vi "AIT 664 - Read incoming message data.vi"(0 "Driver Data":T1 {"Num Bits" min=1 max=32}, 5 "Default Msg Data":u8[](array[numeric]), 11 "error in (no error)":errorcluster) -> (4 "Values":dbl[](array[numeric]), 15 "error out":errorcluster)   [LabVIEW 2013, in "AIT 664 Custom Device.lvlib"]
doc: "Given channel definition convert U8 data from AIT 664 card to double array that can then be sent to Veristand"
uses:
  AIT 664 Custom Device.lvlib
  RT Controls/AIT 664 - Driver Data.ctl
  Controls and Global/Start Bit.ctl
  Controls and Global/Number of Bits.ctl
  System Explorer/Controls/664 -Param.ctl
  <vilib>/NI Veristand/Custom Device Tools/Custom Device Utility Library/Custom Device Utility Library.lvlib
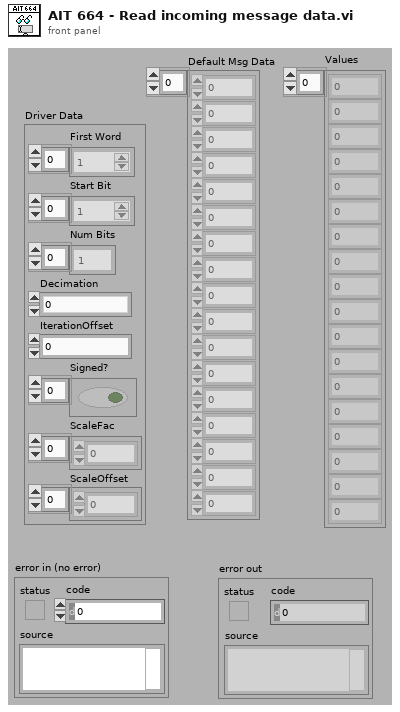
[diagram p1: front panel]
types:
  T1 = typedef "AIT 664 Custom Device.lvlib/AIT 664 - Driver Data.ctl" = cluster{"First Word":T2[], "Start Bit":T2[], "Num Bits":T3[], "Decimation":i32, "IterationOffset":i32, "Signed?":bool[], "ScaleFac":dbl[], "ScaleOffset":dbl[]}
  T2 = typedef "AIT 664 Custom Device.lvlib/Start Bit.ctl" = i32
  T3 = typedef "AIT 664 Custom Device.lvlib/Number of Bits.ctl" = i32
  T4 = typedef "AIT 664 Custom Device.lvlib/664 -Param.ctl" = cluster{"name":string, "firstByte":i32, "startBit":i32, "numberBits":i32, "scaleFactor":dbl, "scaleOffset":dbl, "signed":bool}
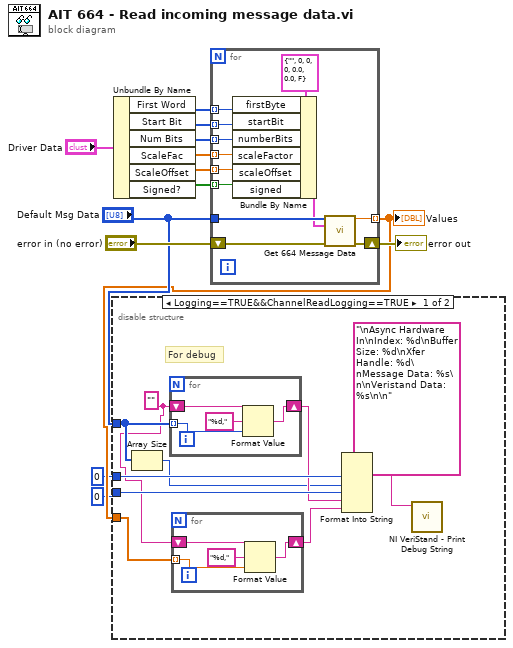
[diagram p0: block diagram]
diagram:
  n1 = Unbundle By Name("Driver Data") -> ("First Word"=w11:T2[], "Start Bit"=w10:T2[], "Num Bits"=w9:T3[], "ScaleFac"=w8:dbl[], "ScaleOffset"=w7:dbl[], "Signed?"=w6:bool[])
  n2 = for {
    tunnel: "Default Msg Data" -> [w25]
    tunnel: w11 -> [w22] mode=indexing
    tunnel: w10 -> [w21] mode=indexing
    tunnel: w9 -> [w20] mode=indexing
    tunnel: w8 -> [w19] mode=indexing
    tunnel: w7 -> [w18] mode=indexing
    tunnel: w6 -> [w17] mode=indexing
    tunnel: [w15] -> w3 mode=indexing
    shift-right: [w14] -> w5
    shift-left: "error in (no error)" -> [w24]
    n3 = Bundle By Name(cluster=T4 {"name"="", "firstByte"=0, "startBit"=0, "numberBits"=0, "scaleFactor"=0.0, "scaleOffset"=0.0, "signed"=FALSE} ("1553 Parameter"), "firstByte"=w22, "startBit"=w21, "numberBits"=w20, "scaleFactor"=w19, "scaleOffset"=w18, "signed"=w17) -> (w16:T4)
    n4 = call "Get 664 Message Data.vi"("MSG DATA"=w25, "664 Parameter"=w16, "error in (no error)"=w24) -> ("Value"=w15:dbl, "error out"=w14:errorcluster)  [unwired: 11 in]
  }
  "error out" <- w5
  "Values" <- w3
  n5 = disable-structure shown="Logging==TRUE&&ChannelReadLogging==TRUE" {
    disable-tunnel: "Default Msg Data" -> [w30 _]
    disable-tunnel: 0 ("Channel Index") -> [w35 _]
    disable-tunnel: 0 ("Decimation") -> [w34 _]
    disable-tunnel: w3 -> [w28 _]
    frame condition #0 (active) {
      w27 = "" ("format string")
      # "For debug"
      n6 = Array Size(array=w30) -> (size(s)=w29:i32)
      n7 = for {
        tunnel: w30 -> [w40] mode=indexing
        shift-right: [w41] -> w32
        shift-left: w27 -> [w42]
        n8 = Format Value(string ("")=w42, format string="%d,", value (0)=w40) -> (output string=w41:string)
      }
      n9 = for {
        tunnel: w28 -> [w36] mode=indexing
        shift-right: [w37] -> w26
        shift-left: w27 -> [w38]
        n10 = Format Value(string ("")=w38, format string="%d,", value (0)=w36) -> (output string=w37:string)
      }
      n11 = Format Into String(format string="\nAsync Hardware In\nIndex: %d\nBuffer Size: %d\nXfer Handle: %d\nMessage Data: %s\n\nVeristand Data: %s\n\n", w35, w29, w34, w32, w26) -> (resulting string=w31:string)  [unwired: 2 in, 1 out]
      n12 = call <vilib>:"NI VeriStand - Print Debug String.vi"("Message"=w31) -> ()  [unwired: 10 in, 1 out]
    }
    frame condition #1 {
    }
  }
